vi "SaveDataInCloud.vi"(9 "DataToBeStored":string, 10 "FileName":string, 11 "CloudAddress":string) -> ()   [LabVIEW 2017]
uses:
  <vilib>/httpClient/PUTBuffer.vi
  <vilib>/httpClient/LabVIEWHTTPClient.lvlib
panel:
  out "concatenated string":string
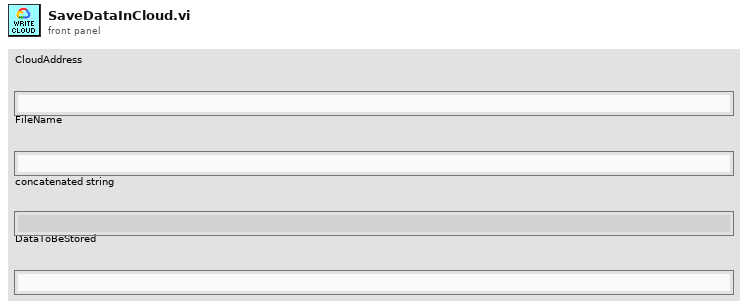
[diagram p1: front panel]
types:
  T1 = typedef "LabVIEWHTTPClient.lvlib/ClientHandle.ctl" = refnum<k1>
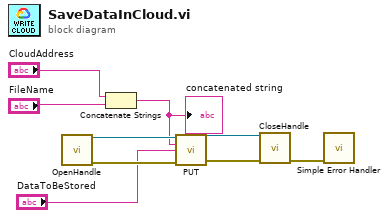
[diagram p0: block diagram]
diagram:
  n1 = call <vilib>:"OpenHandle.vi"() -> ("client handle out"=w9:T1, "error out"=w8:errorcluster)  [unwired: 14 in]
  n2 = Concatenate Strings("CloudAddress", "FileName") -> (w7:string)
  "concatenated string" <- w7
  n3 = call-poly <vilib>:"PUT.vi"("client handle"=w9, "url"=w7, "buffer"="DataToBeStored", "error in (no error)"=w8) -> ("client handle out"=w3:T1, "error out"=w2:errorcluster)  [unwired: 8 in, 2 out]
  n4 = call <vilib>:"CloseHandle.vi"("client handle"=w3, "error in (no error)"=w2) -> ("error out"=w1:errorcluster)  [unwired: 13 in]
  n5 = call <vilib>:"Simple Error Handler.vi"("error in (no error)"=w1) -> ()  [unwired: 4 in, 5 out]
